vi "EnableVision.vi"(7 "Update":bool, 8 "VisionButton":bool, 11 "EnableVision":bool) -> (0 "VisionButtonOut":bool, 3 "EnableVisionOut":bool)   [LabVIEW 2016]
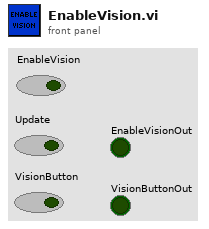
[diagram p1: front panel]
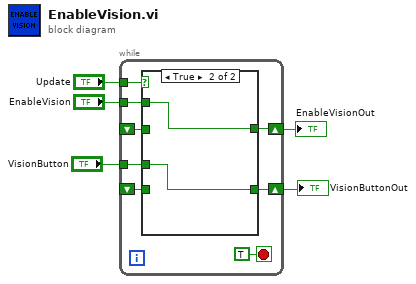
[diagram p0: block diagram]
diagram:
  n1 = while {
    tunnel: "Update" -> [w12]
    tunnel: "EnableVision" -> [w11]
    shift-right: [w10] -> w3
    shift-left: _ -> [w9]
    tunnel: "VisionButton" -> [w8]
    shift-right: [w7] -> w1
    shift-left: _ -> [w6]
    stop <- TRUE stop-if-true
    n2 = case shown="True" w12 {
      tunnel: [w15 w17] -> w10
      tunnel: w11 -> [_ w17]
      tunnel: w9 -> [w15 _]
      tunnel: w8 -> [_ w16]
      tunnel: [w14 w16] -> w7
      tunnel: w6 -> [w14 _]
      frame False {
      }
      frame True {
      }
    }
  }
  "EnableVisionOut" <- w3
  "VisionButtonOut" <- w1
